vi "JVT-Test.vi"() -> ()   [LabVIEW 2009]
uses:
  Support Files/Address.ctl
  <vilib>/Platform/TimedLoop/XDataNode/XDataNode.xnode
  <vilib>/Platform/TimedLoop/XDataNode/loadlvalarms.vi
  <vilib>/Platform/TimedLoop/XDataNode/timing_clust.ctl
  <vilib>/Platform/TimedLoop/XDataNode/nitl_modes.ctl
  <vilib>/Platform/TimedLoop/XDataNode/wakeup.ctl
  <vilib>/Platform/TimedLoop/XDataNode/XDNodeRunTimeDep.lvlib
panel:
  out "Encoded JAUS Message":string
  out "Receive HB":bool
  out "Send HB":bool
  out "Timed out?":bool=TRUE
  out "port":u16
  out "address":u32
  out "received":string
  in  "stop":bool
  in  "Destination":T1={"Subsystem Id"=42, "Node Id"=1, "Component Id"=1}
  in  "Source":T1={"Subsystem Id"=3, "Node Id"=1, "Component Id"=1}
  out "port selected":u16=3794
  in  "Server IP":string="24.42.140.203"
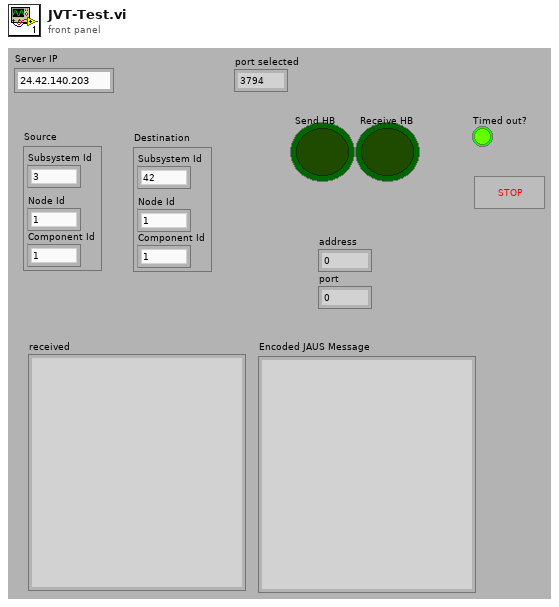
[diagram p1: front panel]
types:
  T1 = typedef "Address.ctl" = cluster{"Subsystem Id":u16, "Node Id":u8, "Component Id":u8}
  T2 = typedef "XDNodeRunTimeDep.lvlib/timing_clust.ctl" = cluster{"Expected End [f-1]":u64, "Actual End [f-1]":u64, "Finished Late? [f-1]":bool, "Expected End [i-1]":u64, "Actual End [i-1]":u64, "Finished Late? [i-1]":bool, "Expected Start [i]":u64, "Actual Start [i]":u64, "Expected Start [f]":u64, "Actual Start [f]":u64, "Source Name":string, "Structure Name":string, "Period":i64, "Deadline":i64, "Offset":i64, "Start":i64, "Priority":i32, "Timeout":i32, "Mode":T3, "Wakeup Reason":T4, "Error":errorcluster, "Source Type":string, "Secondary Source Type":string, "Global End Time":u64, "Global Start Time":u64, "Frame Duration":u64, "Iteration Duration":u64, "Assigned CPU":i32, "I/O Scan Engine Mode":u32}
  T3 = typedef "XDNodeRunTimeDep.lvlib/nitl_modes.ctl" = enum32{"No Change", "Process missed periods, maintain original phase", "Discard missed periods, maintain original phase", "Process missed periods, ignore original phase", "Discard missed periods, ignore original phase"}
  T4 = typedef "XDNodeRunTimeDep.lvlib/wakeup.ctl" = enum32{"Normal", "Aborted", "Asynchronous wakeup", "Timing source error", "Timed loop error", "Timeout"}
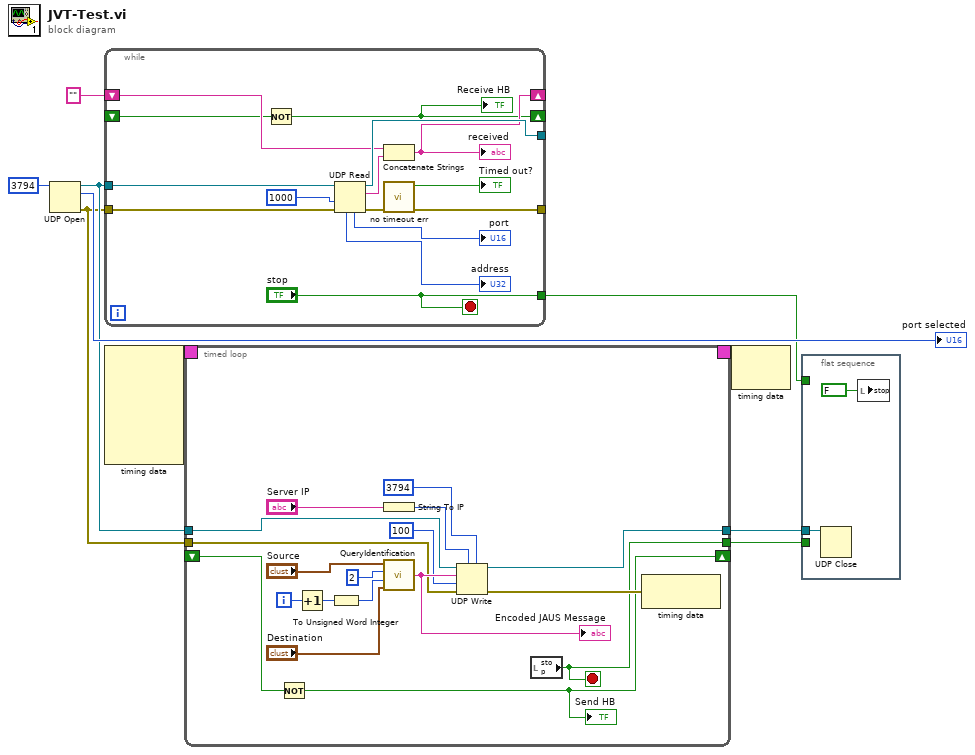
[diagram p0: block diagram]
diagram:
  n1 = UDP Open(11:u16 3794 ("port")) -> (port=w9:refnum<k16>, 0:w8:errorcluster, 2:→"port selected":u16)  [unwired: 4 in]
  n2 = while {
    tunnel: w9 -> [w25]
    tunnel: [w24] -> _
    tunnel: w8 -> [w20]
    tunnel: [w18] -> _
    tunnel: ["stop"] -> w3
    shift-right: [w14] -> _
    shift-left: "" -> [w16]
    shift-right: [w11] -> _
    shift-left: _ -> [w12]
    stop <- "stop" stop-if-true
    n3 = Not(x=w12) -> (.not. x?=w11:bool)
    "Receive HB" <- w11
    n4 = UDP Read(connection ID=w25, timeout ms (25000)=1000, 8:w20) -> (data out=w15:string, error out=w19:errorcluster, 3:w24:refnum<k16>, 4:→"port":u16, 6:→"address":u32)  [unwired: 1 in]
    n5 = Concatenate Strings(w16, w15) -> (w14:string)
    "received" <- w14
    n6 = call "no timeout err.vi"("error in (no error)"=w19) -> ("error out"=w18:errorcluster, "Timed out?"=→"Timed out?":bool)  [unwired: 9 in]
  }
  n7 = node-c288() -> (w7:T2)  [unwired: 6 in]
  n8 = timed-loop {
    timing: w7 -> [_]
    timing-out: [_] -> w6
    tunnel: w9 -> [w43]
    tunnel: [w40] -> w2
    tunnel: w8 -> [w37]
    tunnel: [w32] -> w4
    shift-right: [w26] -> _
    shift-left: _ -> [w27]
    i -> [w31]
    stop <- w32 stop-if-true
    n9 = Not(x=w27) -> (.not. x?=w26:bool)
    "Send HB" <- w26
    n10 = Increment(x=w31) -> (x+1=w30:i32)
    n11 = To Unsigned Word Integer(number=w30) -> (unsigned 16bit integer=w29:u16)
    n12 = String To IP(1:"Server IP") -> (0:w41:u32)
    n13 = call "QueryIdentification.vi"("Destination"="Destination", "Sequence Number (16 bits)"=w29, "QueryType"=u8 2, "Source"="Source") -> ("Encoded JAUS Message"=w39:string)
    "Encoded JAUS Message" <- w39
    n14 = UDP Write(address=w41, port or service name=u16 3794 ("Port"), connection ID=w43, data in=w39, 8:w37, 9:100 ("timeout ms (25000)")) -> (error out=w42:errorcluster, 3:w40:refnum<k16>)
    n15 = local read "stop"() -> (w32:bool)
    n16 = node-c288(w42) -> ()  [unwired: 1 out]
  }
  n17 = node-c288(w6) -> ()  [unwired: 1 out]
  n18 = flat-sequence {
    tunnel: w4 -> [_]
    tunnel: w3 -> [_]
    tunnel: w2 -> [w48]
    frame #0 {
      n19 = UDP Close(connection ID=w48) -> ()  [unwired: 1 in, 2 out]
      n20 = local write "stop"(FALSE ("stop")) -> ()
    }
  }
